vi "_RT_Init_MemoryConfiguration.vi"(8 "error in (no error)":errorcluster) -> (0 "error out":errorcluster, 1 "RT_SysTimeStamp":timestamp, 2 "system state":refnum<data-value>, 3 "Signal Queue":refnum<queue>)   [LabVIEW 2018]
uses:
  PublicSubVI/Ctl/_ctl_RT_System_State.ctl
  PublicSubVI/Ctl/_ctl_RT_NS_Status.ctl
  PublicSubVI/Ctl/_ctl_RT_TurboSettings.ctl
  PC/Daemon/RecipeEditor/Ctl/WfmCmd_Type.ctl
  ControlLoop/Laser/Ctl/_ctl_LaserParam.ctl
  PublicSubVI/Ctl/_ctl_Integrated_Cmd.ctl
  PublicSubVI/Ctl/_ctl_RT_ExtAO.ctl
  PublicSubVI/Ctl/_ctl_RT_extDO.ctl
  PublicSubVI/Ctl/_ctl_RT_D999_Format.ctl
  PublicSubVI/Ctl/_ctl_RT_D999_Param.ctl
  PublicSubVI/Ctl/_ctl_RT_Working_State.ctl
  PublicSubVI/Ctl/_ctl_RT_D999_Command.ctl
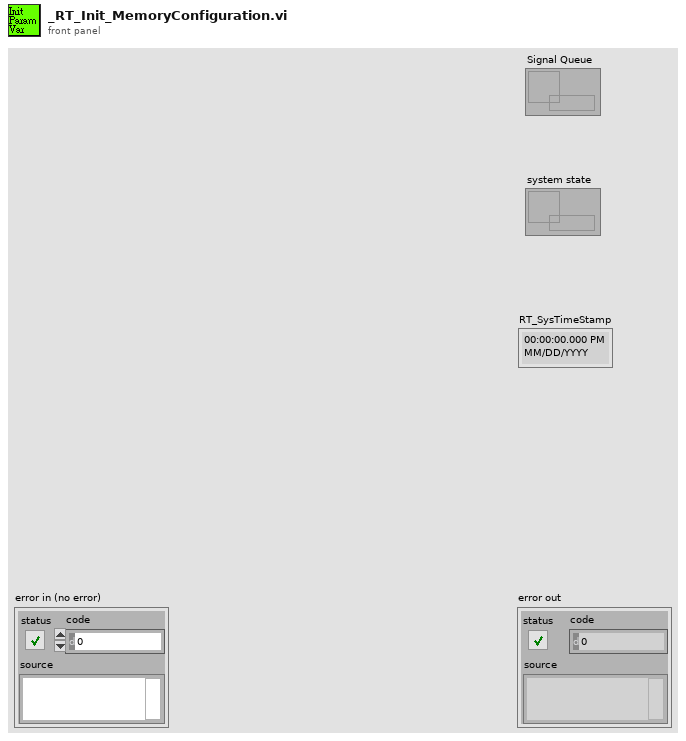
[diagram p1: front panel]
types:
  T1 = typedef "_ctl_RT_D999_Command.ctl" = cluster{"label":string, "value":variant}
  T2 = typedef "_ctl_RT_Working_State.ctl" = enum16{"Initialize", "Running", "Reboot_Work", "Reboot_Safe"}
  T3 = typedef "_ctl_RT_System_State.ctl" = enum16{"initialize", "idle", "working", "disconnect"}
  T4 = typedef "_ctl_RT_D999_Param.ctl" = cluster{"Enable":bool, "AI":cluster{"Label":string, "MultiValue":dbl, "AddValue":dbl}[], "AO":i16[], "Switch":bool[]}
  T5 = typedef "_ctl_RT_extDO.ctl" = cluster{"Label":string, "Boolean":bool}[]
  T6 = typedef "_ctl_RT_D999_Format.ctl" = cluster{"Port":string, "Label":string, "Value":dbl}[]
  T7 = typedef "_ctl_RT_ExtAO.ctl" = cluster{"Label":string, "y":dbl}[]
  T8 = typedef "_ctl_Integrated_Cmd.ctl" = enum8{"Init", "Set", "Get", "Read", "Write", "Send", "Idle", "Startup", "Execution", "End", "Close"}
  T9 = typedef "WfmCmd_Type.ctl" = enum8{"None", "WFM", "EventCodes"}
  T10 = typedef "_ctl_LaserParam.ctl" = cluster{"Energy":dbl, "Freq":dbl, "Emission":bool, "TriggerSource":enum16{"Internal", "External"}, "Time Stamp":timestamp}
  T11 = typedef "_ctl_RT_TurboSettings.ctl" = cluster{"Preset rot. speed \nat standby mode(%)":dbl, "Speed set value in rot. speed \nsetting operations (%)":dbl, "Max. power (%)":dbl, "Gas mode: ":enum16{"heavy", "light", "helium"}, "Operations mode: ":bool, "Motor turbopump: ":bool, "Pumping station: ":bool, "Standby: ":bool, "Timestamp":timestamp}
  T12 = cluster{"AI 0":fxp<+/-,24,5>, "AI 1":fxp<+/-,24,5>, "AI 2":fxp<+/-,24,5>, "AI 3":fxp<+/-,24,5>, "AI 4":fxp<+/-,24,5>, "AI 5":fxp<+/-,24,5>, "AI 6":fxp<+/-,24,5>, "AI 7":fxp<+/-,24,5>, "AI 8":fxp<+/-,24,5>, "AI 9":fxp<+/-,24,5>, "AI 10":fxp<+/-,24,5>, "AI 11":fxp<+/-,24,5>, "AI 12":fxp<+/-,24,5>, "AI 13":fxp<+/-,24,5>, "AI 14":fxp<+/-,24,5>, "AI 15":fxp<+/-,24,5>}
  T13 = typedef "_ctl_RT_NS_Status.ctl" = enum8{"Idle", "Init", "Connected", "Stop"}
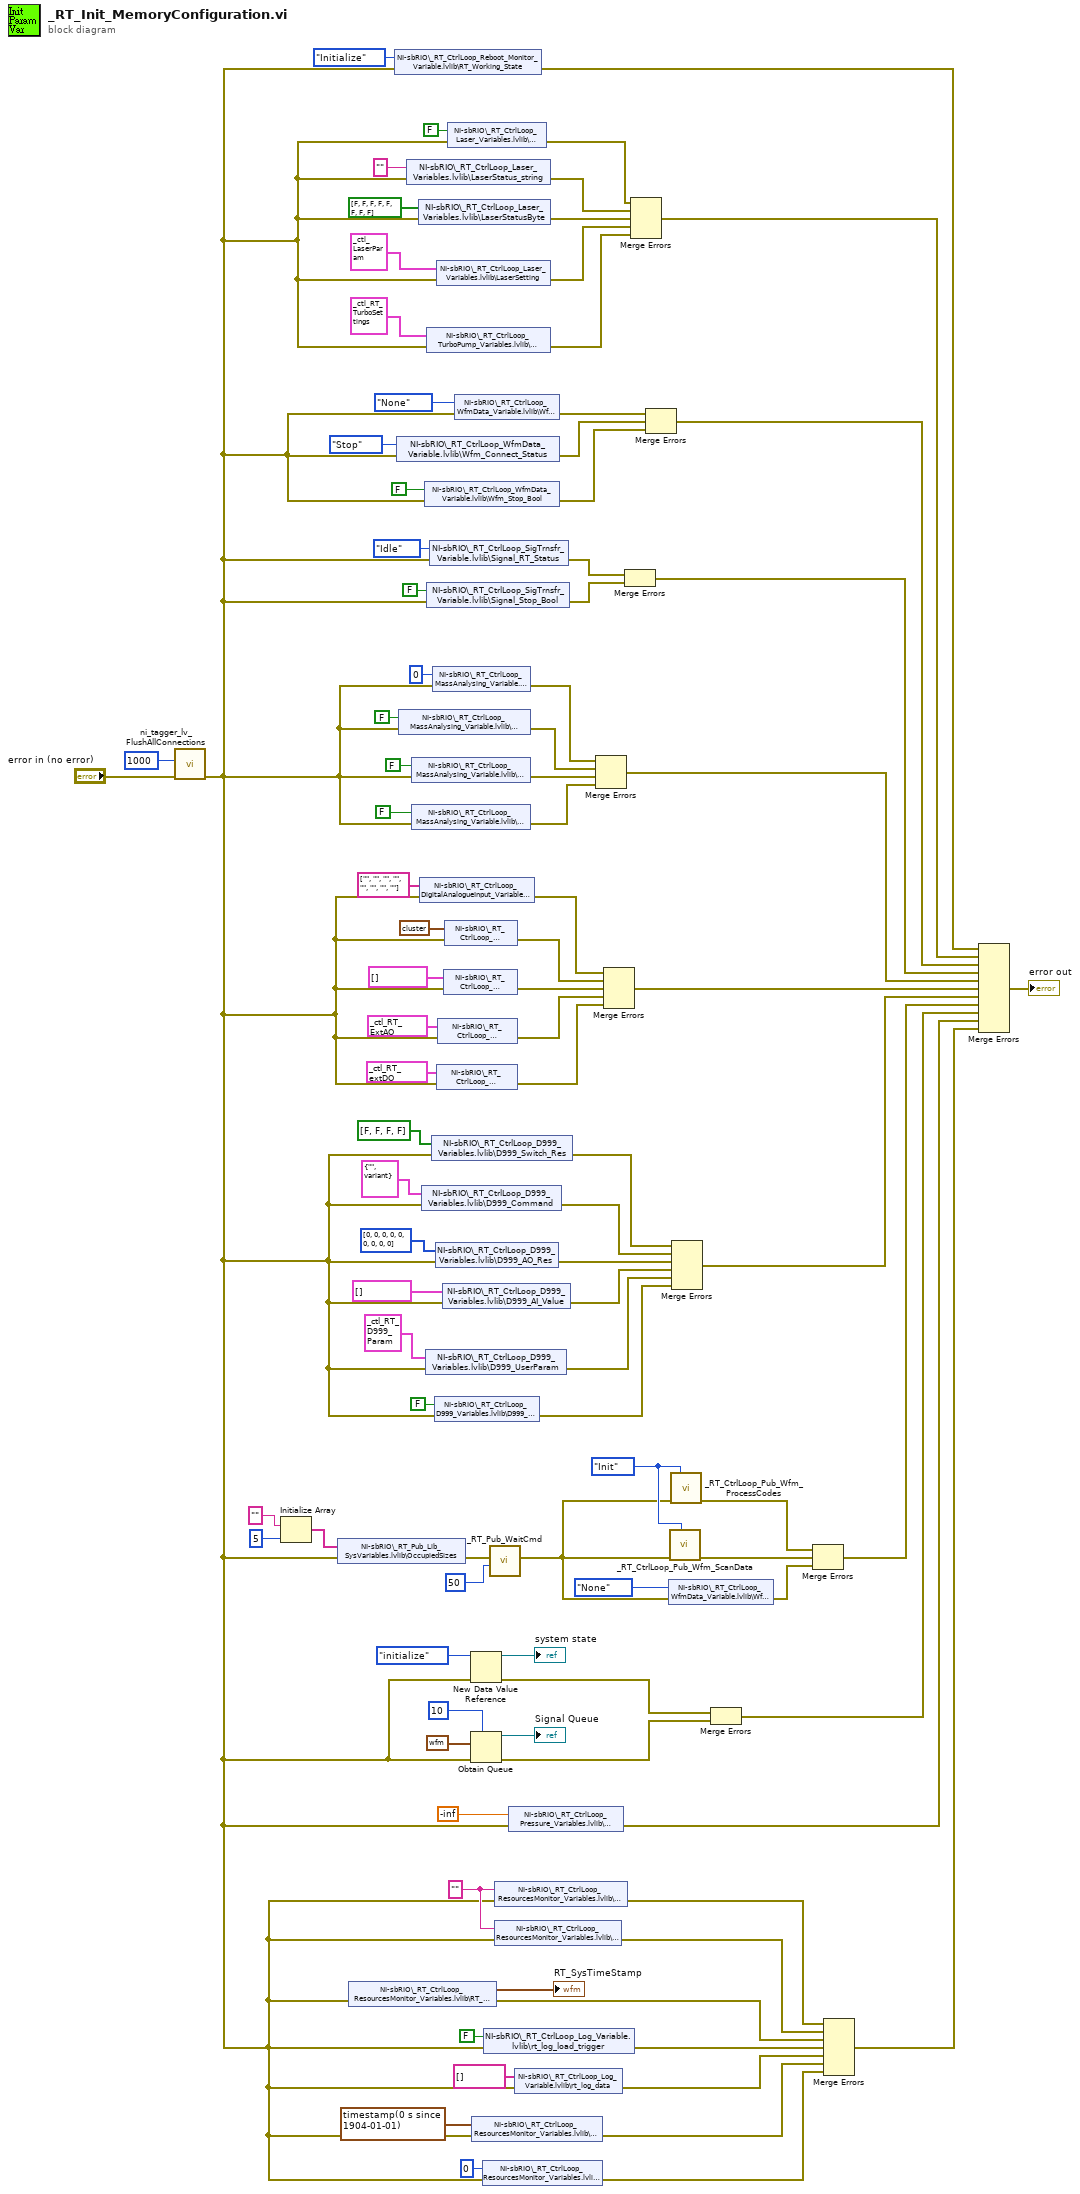
[diagram p0: block diagram]
diagram:
  w44 = "" ("ResourceUsage")
  w82 = _ctl_Integrated_Cmd."Init" ("Enum")
  n1 = call <vilib>:"ni_tagger_lv_FlushAllConnections.vi"("error in (no error)"="error in (no error)", "timeout ms (1000)"=1000) -> ("error out"=w2:errorcluster)  [unwired: 8 in, 1 out]
  n2 = Initialize Array("", 5 ("dimension size")) -> (w97:string[])
  n3 = shared-variable "NI-sbRIO\\_RT_Pub_Lib_SysVariables.lvlib\\OccupiedSizes"(w97, error in=w2) -> (error out=w78:errorcluster)
  n4 = shared-variable "NI-sbRIO\\_RT_CtrlLoop_ResourcesMonitor_Variables.lvlib\\RT_SysTimeStamp"(error in=w2) -> (→"RT_SysTimeStamp":timestamp, error out=w18:errorcluster)
  n5 = shared-variable "NI-sbRIO\\_RT_CtrlLoop_Reboot_Monitor_Variable.lvlib\\RT_Working_State"(_ctl_RT_Working_State."Initialize" ("RT_Working_State"), error in=w2) -> (error out=w1:errorcluster)
  n6 = shared-variable "NI-sbRIO\\_RT_CtrlLoop_WfmData_Variable.lvlib\\Wfm_Connect_Status"(_ctl_RT_NS_Status."Stop" ("Wfm_Connect_Status"), error in=w2) -> (error out=w62:errorcluster)
  n7 = shared-variable "NI-sbRIO\\_RT_CtrlLoop_MassAnalysing_Variable.lvlib\\MassAnalPause"(FALSE ("MassAnalPause"), error in=w2) -> (error out=w71:errorcluster)
  n8 = shared-variable "NI-sbRIO\\_RT_CtrlLoop_Laser_Variables.lvlib\\LaserStatus_string"("" ("LaserStatus_string"), error in=w2) -> (error out=w61:errorcluster)
  n9 = shared-variable "NI-sbRIO\\_RT_CtrlLoop_MassAnalysing_Variable.lvlib\\MassAnalExe"(FALSE ("MassAnalExe"), error in=w2) -> (error out=w70:errorcluster)
  n10 = shared-variable "NI-sbRIO\\_RT_CtrlLoop_MassAnalysing_Variable.lvlib\\MassAnalExe"(FALSE ("MassAnalEnable"), error in=w2) -> (error out=w33:errorcluster)
  n11 = shared-variable "NI-sbRIO\\_RT_CtrlLoop_Laser_Variables.lvlib\\LaserStatusByte"(bool[] [FALSE, FALSE, FALSE, FALSE, FALSE, FALSE, FALSE, FALSE] ("LaserStatusByte"), error in=w2) -> (error out=w60:errorcluster)
  n12 = shared-variable "NI-sbRIO\\_RT_CtrlLoop_DigitalAnalogueInput_Variables.lvlib\\ExtDI_Labels"(string[] ["", "", "", "", "", "", "", ""], error in=w2) -> (error out=w36:errorcluster)
  n13 = shared-variable "NI-sbRIO\\_RT_CtrlLoop_D999_Variables.lvlib\\D999_Command"(T1 {"label"="", "value"=variant} ("D999_Command"), error in=w2) -> (error out=w4:errorcluster)
  n14 = shared-variable "NI-sbRIO\\_RT_CtrlLoop_WfmData_Variable.lvlib\\Wfm_Stop_Bool"(FALSE ("Wfm_Stop_Bool"), error in=w2) -> (error out=w21:errorcluster)
  n15 = shared-variable "NI-sbRIO\\_RT_CtrlLoop_D999_Variables.lvlib\\D999_UserParam"(T4 {"Enable"=FALSE, "AI"=[{"Label"="", "MultiValue"=1.0, "AddValue"=0.0}, {"Label"="", "MultiValue"=1.0, "AddValue"=0.0}, {"Label"="", "MultiValue"=1.0, "AddValue"=0.0}, {"Label"="", "MultiValue"=1.0, "AddValue"=0.0}, {"Label"="", "MultiValue"=1.0, "AddValue"=0.0}, {"Label"="", "MultiValue"=1.0, "AddValue"=0.0}, {"Label"="", "MultiValue"=1.0, "AddValue"=0.0}, {"Label"="", "MultiValue"=1.0, "AddValue"=0.0}, {"Label"="", "MultiValue"=1.0, "AddValue"=0.0}, {"Label"="", "MultiValue"=1.0, "AddValue"=0.0}, {"Label"="", "MultiValue"=1.0, "AddValue"=0.0}, {"Label"="", "MultiValue"=1.0, "AddValue"=0.0}], "AO"=[], "Switch"=[]} ("D999_AI_Param"), error in=w2) -> (error out=w39:errorcluster)
  n16 = shared-variable "NI-sbRIO\\_RT_CtrlLoop_TurboPump_Variables.lvlib\\TurboSettings"(T11 {"Preset rot. speed \nat standby mode(%)"=0.0, "Speed set value in rot. speed \nsetting operations (%)"=0.0, "Max. power (%)"=0.0, "Gas mode: "=enum."heavy", "Operations mode: "=FALSE, "Motor turbopump: "=FALSE, "Pumping station: "=FALSE, "Standby: "=FALSE, "Timestamp"=timestamp(0 s since 1904-01-01)} ("TurboSettings"), error in=w2) -> (error out=w58:errorcluster)
  n17 = shared-variable "NI-sbRIO\\_RT_CtrlLoop_SigTrnsfr_Variable.lvlib\\Signal_Stop_Bool"(FALSE ("Signal_Stop_Bool"), error in=w2) -> (error out=w49:errorcluster)
  n18 = shared-variable "NI-sbRIO\\_RT_CtrlLoop_SigTrnsfr_Variable.lvlib\\Signal_RT_Status"(enum8{"Idle", "Init", "Connected", "Stop"}."Idle" ("Signal_RT_Status"), error in=w2) -> (error out=w50:errorcluster)
  n19 = shared-variable "NI-sbRIO\\_RT_CtrlLoop_D999_Variables.lvlib\\D999_Switch_Res"(bool[] [FALSE, FALSE, FALSE, FALSE] ("D999_Switch_Res"), error in=w2) -> (error out=w30:errorcluster)
  n20 = shared-variable "NI-sbRIO\\_RT_CtrlLoop_MassAnalysing_Variable.lvlib\\ExeTimes"(0 ("ExeTimes"), error in=w2) -> (error out=w72:errorcluster)
  n21 = shared-variable "NI-sbRIO\\_RT_CtrlLoop_D999_Variables.lvlib\\D999_Exist"(FALSE ("D999_Exist"), error in=w2) -> (error out=w15:errorcluster)
  n22 = shared-variable "NI-sbRIO\\_RT_CtrlLoop_D999_Variables.lvlib\\D999_AO_Res"(i16[] [0, 0, 0, 0, 0, 0, 0, 0, 0] ("D999_AO_Res"), error in=w2) -> (error out=w55:errorcluster)
  n23 = shared-variable "NI-sbRIO\\_RT_CtrlLoop_Laser_Variables.lvlib\\LaserSetting"(T10 {"Energy"=50.0, "Freq"=0.0, "Emission"=FALSE, "TriggerSource"=enum."External", "Time Stamp"=timestamp(0 s since 1904-01-01)} ("_cluster_Laser349"), error in=w2) -> (error out=w59:errorcluster)
  n24 = shared-variable "NI-sbRIO\\_RT_CtrlLoop_DigitalAnalogueOutput_Variables.lvlib\\ExtDO"(T5 [{"Label"="", "Boolean"=FALSE}, {"Label"="", "Boolean"=FALSE}, {"Label"="", "Boolean"=FALSE}, {"Label"="", "Boolean"=FALSE}, {"Label"="", "Boolean"=FALSE}, {"Label"="", "Boolean"=FALSE}, {"Label"="", "Boolean"=FALSE}, {"Label"="", "Boolean"=FALSE}] ("ExtDO"), error in=w2) -> (error out=w64:errorcluster)
  n25 = shared-variable "NI-sbRIO\\_RT_CtrlLoop_DigitalAnalogueOutput_Variables.lvlib\\ExtAO"(T7 [{"Label"="", "y"=0.0}, {"Label"="", "y"=0.0}, {"Label"="", "y"=0.0}, {"Label"="", "y"=0.0}, {"Label"="", "y"=0.0}, {"Label"="", "y"=0.0}, {"Label"="", "y"=0.0}, {"Label"="", "y"=0.0}] ("ExtAO"), error in=w2) -> (error out=w65:errorcluster)
  n26 = shared-variable "NI-sbRIO\\_RT_CtrlLoop_D999_Variables.lvlib\\D999_AI_Value"(T6 [] ("EC_AllValue"), error in=w2) -> (error out=w54:errorcluster)
  n27 = shared-variable "NI-sbRIO\\_RT_CtrlLoop_DigitalAnalogueInput_Variables.lvlib\\ExtDI"(T5 [] ("DI in"), error in=w2) -> (error out=w66:errorcluster)
  n28 = shared-variable "NI-sbRIO\\_RT_CtrlLoop_DigitalAnalogueInput_Variables.lvlib\\ExtAI"(T12 {"AI 0"=0.0, "AI 1"=0.0, "AI 2"=0.0, "AI 3"=0.0, "AI 4"=0.0, "AI 5"=0.0, "AI 6"=0.0, "AI 7"=0.0, "AI 8"=0.0, "AI 9"=0.0, "AI 10"=0.0, "AI 11"=0.0, "AI 12"=0.0, "AI 13"=0.0, "AI 14"=0.0, "AI 15"=0.0} ("ExtAI"), error in=w2) -> (error out=w67:errorcluster)
  n29 = shared-variable "NI-sbRIO\\_RT_CtrlLoop_Laser_Variables.lvlib\\LaserExist"(FALSE ("LaserExist"), error in=w2) -> (error out=w19:errorcluster)
  n30 = shared-variable "NI-sbRIO\\_RT_CtrlLoop_WfmData_Variable.lvlib\\Wfm_Type"(WfmCmd_Type."None" ("Wfm_Type"), error in=w2) -> (error out=w63:errorcluster)
  n31 = New Data Value Reference ("system state")(data value=_ctl_RT_System_State."initialize" ("system_state"), error in=w2) -> (data value reference=→"system state":refnum<data-value>, error out=w27:errorcluster)
  n32 = Obtain Queue(max queue size (-1, unlimited)=10, element data type=waveform(i16) {"t0"=timestamp(0 s since 1904-01-01), "dt"=1.0, "Y"=[]} ("element"), error in (no error)=w2) -> (queue out=→"Signal Queue":refnum<queue>, error out=w57:errorcluster)  [unwired: 2 in, 1 out]
  n33 = shared-variable "NI-sbRIO\\_RT_CtrlLoop_ResourcesMonitor_Variables.lvlib\\RT_timeupdate"(timestamp(0 s since 1904-01-01) ("RT_timeupdate"), error in=w2) -> (error out=w14:errorcluster)
  n34 = shared-variable "NI-sbRIO\\_RT_CtrlLoop_ResourcesMonitor_Variables.lvlib\\RT TimeZone"(0 ("RT TimeZone"), error in=w2) -> (error out=w11:errorcluster)
  n35 = shared-variable "NI-sbRIO\\_RT_CtrlLoop_Log_Variable.lvlib\\rt_log_load_trigger"(FALSE ("load_log_trigger"), error in=w2) -> (error out=w23:errorcluster)
  n36 = call "_RT_Pub_WaitCmd.vi"("milliseconds to wait"=u32 50, "error in (no error)"=w78) -> ("error out"=w77:errorcluster)  [unwired: 9 in]
  n37 = shared-variable "NI-sbRIO\\_RT_CtrlLoop_ResourcesMonitor_Variables.lvlib\\ResourceUsage"(w44, error in=w2) -> (error out=w43:errorcluster)
  n38 = shared-variable "NI-sbRIO\\_RT_CtrlLoop_ResourcesMonitor_Variables.lvlib\\SystemVersion"(w44, error in=w2) -> (error out=w42:errorcluster)
  n39 = shared-variable "NI-sbRIO\\_RT_CtrlLoop_Pressure_Variables.lvlib\\Pressure_dbl"(-inf, error in=w2) -> (error out=w7:errorcluster)
  n40 = shared-variable "NI-sbRIO\\_RT_CtrlLoop_Log_Variable.lvlib\\rt_log_data"(string[] [] ("rt_log_data"), error in=w2) -> (error out=w22:errorcluster)
  n41 = Merge Errors(w72, w71, w70, w33) -> (w56:errorcluster)
  n42 = Merge Errors(w36, w67, w66, w65, w64) -> (w35:errorcluster)
  n43 = Merge Errors(w50, w49) -> (w45:errorcluster)
  n44 = Merge Errors(w19, w61, w60, w59, w58) -> (w47:errorcluster)
  n45 = Merge Errors(w63, w62, w21) -> (w46:errorcluster)
  n46 = shared-variable "NI-sbRIO\\_RT_CtrlLoop_WfmData_Variable.lvlib\\Wfm_Type"(WfmCmd_Type."None" ("Wfm_Value"), error in=w77) -> (error out=w81:errorcluster)
  n47 = call "_RT_CtrlLoop_Pub_Wfm_ScanData.vi"("Function"=w82, "error in (no error)"=w77) -> ("error out"=w80:errorcluster)  [unwired: 8 in, 1 out]
  n48 = call "_RT_CtrlLoop_Pub_Wfm_ProcessCodes.vi"("Function"=w82, "error in (no error)"=w77) -> ("error out"=w79:errorcluster)  [unwired: 6 in, 3 out]
  n49 = Merge Errors(w30, w4, w55, w54, w39, w15) -> (w51:errorcluster)
  n50 = Merge Errors(w27, w57) -> (w53:errorcluster)
  n51 = Merge Errors(w79, w80, w81) -> (w52:errorcluster)
  n52 = Merge Errors(w43, w42, w18, w23, w22, w14, w11) -> (w8:errorcluster)
  n53 = Merge Errors(w1, w47, w46, w45, w56, w35, w51, w52, w53, w7, w8) -> (→"error out":errorcluster)
